vi "Read Configuration.vi"(8 "error in (no error)":errorcluster) -> (0 "error out":errorcluster, 3 "connection string":string)   [LabVIEW 2019, in "LV-Data.PGSQL.lvclass"]
uses:
  LV-Data.PGSQL.lvclass
  <vilib>/Utility/config.llb/NI_LVConfig.lvlib
  <vilib>/Utility/config.llb/Read Key (String).vi
panel:
  out "found?":bool
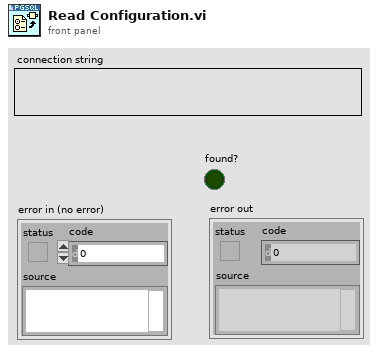
[diagram p1: front panel]
types:
  T1 = typedef "NI_LVConfig.lvlib/Config Data RefNum.ctl" = refnum<k1>
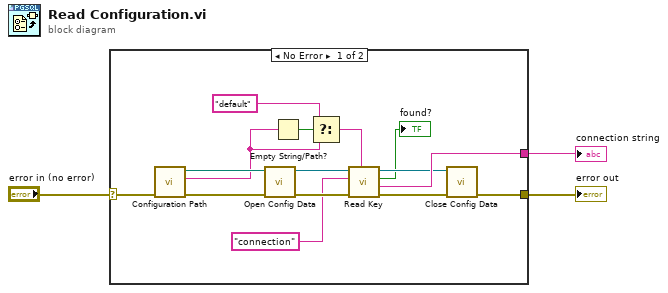
[diagram p0: block diagram]
diagram:
  n1 = case shown="No Error" "error in (no error)" {
    selector: "error in (no error)" -> [w18 w19]
    tunnel: [w17 w19] -> w3
    tunnel: [w16 _] -> w1
    frame No Error {
      n2 = call "Configuration Path.vi"("error in (no error)"=w18) -> ("error out"=w14:errorcluster, "section"=w13:string, "path"=w15:path)  [unwired: 8 in]
      n3 = call <vilib>:"Open Config Data.vi"("error in (no error)"=w14, "configuration file path"=w15) -> ("error out"=w11:errorcluster, "refnum"=w12:T1)  [unwired: 7 in, 1 out]
      n4 = Empty String/Path?(string/path=w13) -> (empty?=w6:bool)
      n5 = Select(t="default" ("section"), s=w6, f=w13) -> (s? t:f=w4:string)
      n6 = call-poly <vilib>:"Read Key.vi"("section"=w4, "error in (no error)"=w11, "key"="connection", "refnum"=w12) -> ("error out"=w10:errorcluster, "value"=w16:string, "found?"=→"found?":bool, "refnum out"=w9:T1)  [unwired: 4 in]
      n7 = call <vilib>:"Close Config Data.vi"("error in (no error)"=w10, "refnum"=w9) -> ("error out"=w17:errorcluster)  [unwired: 8 in, 1 out]
    }
    frame Error {
    }
  }
  "error out" <- w3
  "connection string" <- w1
